vi "DDSSequence_BuildRamp.vi"(6 "Freqeuncy (MHz)":dbl[][](array[numeric]), 7 "Power":dbl[][](array[numeric]), 9 "Channels":T2(ring), 10 "Duration (ms)":dbl[][](array[numeric]), 11 "No of  active time blocks":dbl) -> (3 "appended instruction string":string)   [LabVIEW 2016]
panel:
  out "x/y":dbl
  in  "Ramp duration (us)":dbl=40.0 format="%#_6f"
  out "Step seperation (us)":dbl=0.4
  in  "Step Size":dbl=0.01 format="%#_6f"
  in  "Max Value":dbl=1.0 format="%#_13g"
  in  "Min Value":dbl format="%#_6f"
  in  "Ramp type":enum32{"Frequency", "Phase", "Amplitude"}(ring)=enum."Amplitude"
  in  "Ramp trigger source":T1(ring)=enum."BNC_IN_A_RISING"
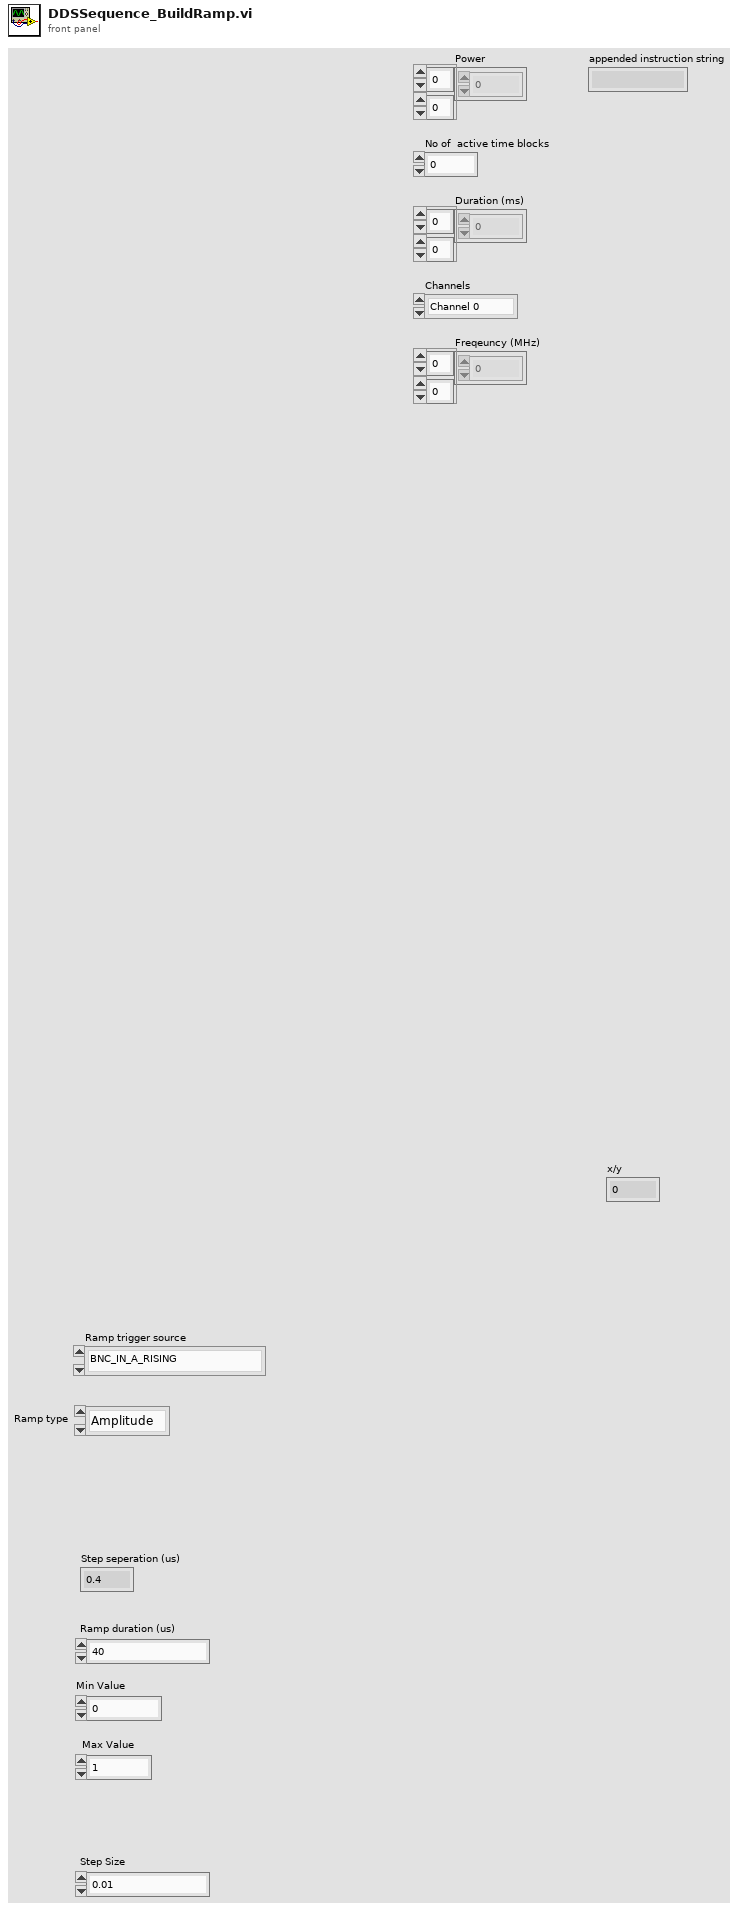
[diagram p1: front panel]
types:
  T1 = enum32{"O_RAMP_SWP_OVR", "RAM_SWP_OVR", "O_DROVER", "DROVER", "O_SPI_FIFO_EV1", "SPI_FIFO_EV1", "O_SPI_FIFO_EV0", "SPI_FIFO_EV0", "O_SPI_FIFO_FLUSHED", "SPI_FIFO_FLUSHED", "BNC_IN_B_LEVEL", "BNC_IN_B_FALLING", "BNC_IN_B_RISING", "BNC_IN_A_LEVEL", "BNC_IN_A_FALLING", "BNC_IN_A_RISING", "ALL_SPI_FIFOS_FLUSHED", "NONE"}
  T2 = enum32{"Channel 0", "Channel 1", "Both channels"}
  T3 = cluster{"Enable ASF from STP (F)":bool, "Digital ramp enable (F)":bool, "Digital ramp no-dwell high (F)":bool, "Digital ramp no-dwell low (F)":bool, "Matched latency enable (T)":bool, "Parallel data port enable (F)":bool}
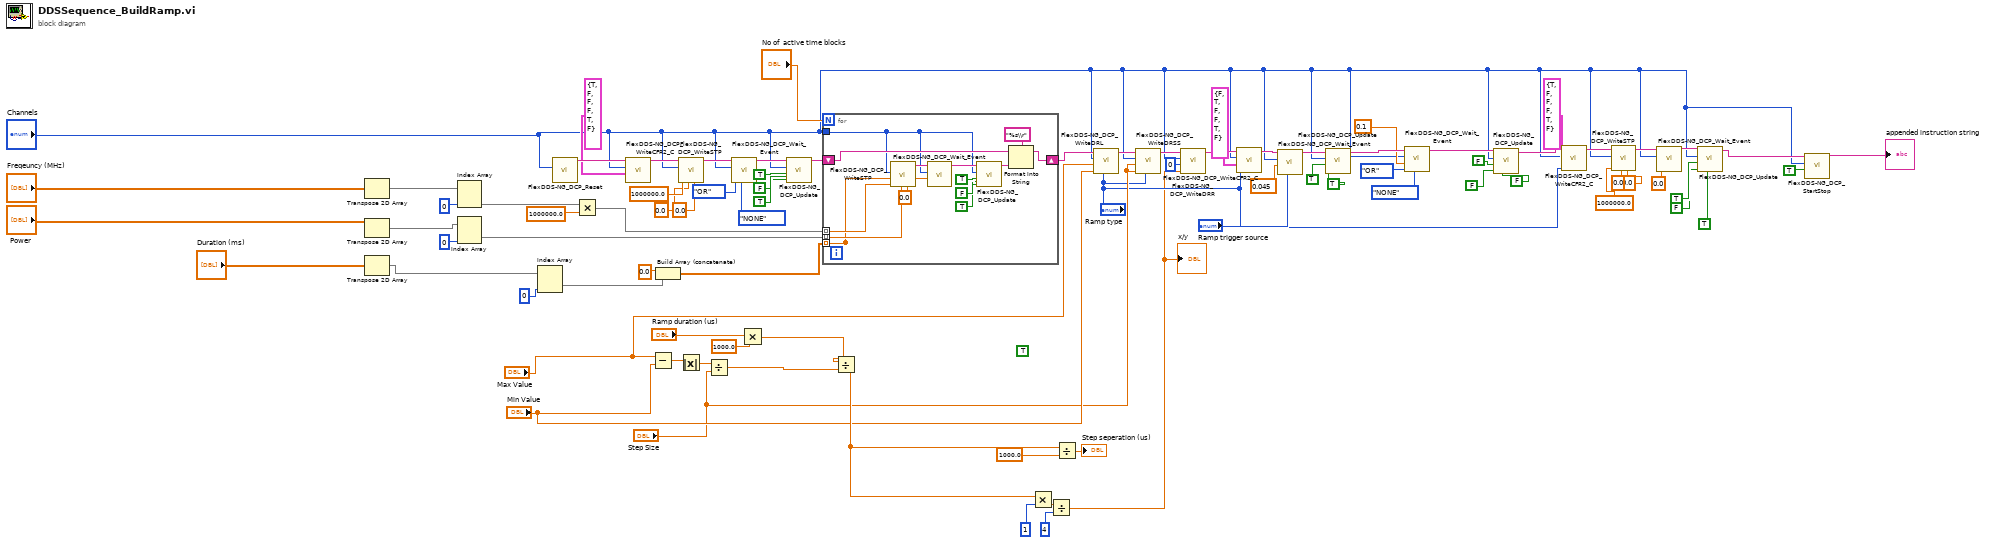
[diagram p0: block diagram]
diagram:
  (unwired) TRUE ("DRCTL(true=+, false=-) 2")
  n1 = Transpose 2D Array(2D array="Freqeuncy (MHz)") -> (transposed array=w74:dbl[][])
  n2 = Transpose 2D Array(2D array="Power") -> (transposed array=w71:dbl[][])
  n3 = Transpose 2D Array(2D array="Duration (ms)") -> (transposed array=w84:dbl[][])
  n4 = Index Array(array=w74, index (col)=0 ("index (row)")) -> (element=w76:dbl[])  [unwired: 1 in]
  n5 = Index Array(array=w71, index (col)=0 ("index (row)")) -> (element=w72:dbl[])  [unwired: 1 in]
  n6 = Index Array(array=w84, index (col)=0 ("index (row)")) -> (element=w81:dbl[])  [unwired: 1 in]
  n7 = call "FlexDDS-NG_DCP_Reset.vi"("Channels"="Channels") -> ("appended instruction string"=w56:string)  [unwired: 10 in]
  n8 = Multiply(x=w76, y=1000000.0 ("frequency Hz (0..400M)")) -> (x*y=w68:dbl[])
  n9 = call "FlexDDS-NG_DCP_WriteCFR2_C.vi"("CFR2 bits"=T3 {"Enable ASF from STP (F)"=TRUE, "Digital ramp enable (F)"=FALSE, "Digital ramp no-dwell high (F)"=FALSE, "Digital ramp no-dwell low (F)"=FALSE, "Matched latency enable (T)"=TRUE, "Parallel data port enable (F)"=FALSE} ("CFR2 bits 2"), "Channels"="Channels", "initial instruction string"=w56) -> ("appended instruction string"=w55:string)  [unwired: 8 in]
  n10 = Subtract(x="Max Value", y="Min Value") -> (x-y=w13:dbl)
  n11 = Build Array (concatenate)(0.0 ("phase degrees (0..360)"), w81) -> (w82:dbl[])
  n12 = call "FlexDDS-NG_DCP_WriteSTP.vi"("phase degrees (0..360)"=0.0, "amplitude (0..1)"=0.0, "frequency Hz (0..400M)"=1000000.0, "Channels"="Channels", "initial instruction string"=w55) -> ("appended instruction string"=w61:string)  [unwired: 6 in]
  n13 = Absolute Value(x=w13) -> (abs(x)=w12:dbl)
  n14 = Divide(x=w12, y="Step Size") -> (x/y=w17:dbl)
  n15 = call "FlexDDS-NG_DCP_Wait_Event.vi"("Event 1"=T1."NONE", "AND/OR"=enum32{"AND", "OR"}."OR", "Channels in"="Channels", "appended instruction string in"=w61) -> ("appended instruction string"=w60:string)  [unwired: 7 in]
  n16 = Multiply(x="Ramp duration (us)", y=1000.0) -> (x*y=w7:dbl)
  n17 = call "FlexDDS-NG_DCP_Update.vi"("ONLY IO_UPDATE"=TRUE, "DRCTL(true=+, false=-)"=FALSE ("DRCTL(true=+, false=-) 2"), "IO_UPDATE(true=u, false = '')"=TRUE ("IO_UPDATE(true=u, false = '')  2"), "Channels"="Channels", "appended instruction string in"=w60) -> ("appended instruction string out"=w66:string)  [unwired: 6 in]
  n18 = for {
    N: "No of  active time blocks" -> [_]
    shift-right: [w90] -> w24
    shift-left: w66 -> [w91]
    tunnel: w72 -> [w88] mode=indexing
    tunnel: "Channels" -> [w87]
    tunnel: w82 -> [w85] mode=indexing
    tunnel: w68 -> [w86] mode=indexing
    tunnel: [w85] -> _ mode=indexing
    n19 = call "FlexDDS-NG_DCP_WriteSTP.vi"("phase degrees (0..360)"=0.0, "amplitude (0..1)"=w88, "frequency Hz (0..400M)"=w86, "Channels"=w87) -> ("appended instruction string"=w93:string)  [unwired: 7 in]
    n20 = call "FlexDDS-NG_DCP_Wait_Event.vi"("waiting time [ms]"=w85, "Channels in"=w87, "appended instruction string in"=w93) -> ("appended instruction string"=w94:string)  [unwired: 8 in]
    n21 = call "FlexDDS-NG_DCP_Update.vi"("ONLY IO_UPDATE"=TRUE, "DRCTL(true=+, false=-)"=FALSE ("DRCTL(true=+, false=-) 2"), "IO_UPDATE(true=u, false = '')"=TRUE ("IO_UPDATE(true=u, false = '')  2"), "Channels"=w87, "appended instruction string in"=w94) -> ("appended instruction string out"=w89:string)  [unwired: 6 in]
    n22 = Format Into String(format string="%s\\r", initial string=w91, w89) -> (resulting string=w90:string)  [unwired: 1 in, 1 out]
  }
  n23 = Divide(x=w7, y=w17) -> (x/y=w16:dbl)
  n24 = Multiply(x=w16, y=u16 1) -> (x*y=w19:dbl)
  n25 = Divide(x=w19, y=u16 4) -> (x/y=w2:dbl)
  "x/y" <- w2
  n26 = Divide(x=w16, y=1000.0 ("x/y")) -> (x/y=→"Step seperation (us)":dbl)
  n27 = call "FlexDDS-NG_DCP_WriteDRL.vi"("Ramp type"="Ramp type", "low limit"="Min Value", "high limit"="Max Value", "Channels"="Channels", "initial instruction string"=w24) -> ("appended instruction string"=w51:string)  [unwired: 6 in]
  n28 = call "FlexDDS-NG_DCP_WriteDRSS.vi"("Ramp type"="Ramp type", "increment step size"="Step Size", "decrement step size"="Step Size", "Channels"="Channels", "initial instruction string"=w51) -> ("appended instruction string"=w50:string)  [unwired: 6 in]
  n29 = call "FlexDDS-NG_DCP_WriteDRR.vi"("digital ramp positive slope rate"=w2, "digital ramp negative slope rate"=u16 0, "Channels"="Channels", "initial instruction string"=w50) -> ("appended instruction string"=w49:string)  [unwired: 7 in]
  n30 = call "FlexDDS-NG_DCP_WriteCFR2_C.vi"("Digital ramp destination"="Ramp type", "CFR2 bits"=T3 {"Enable ASF from STP (F)"=FALSE, "Digital ramp enable (F)"=TRUE, "Digital ramp no-dwell high (F)"=FALSE, "Digital ramp no-dwell low (F)"=FALSE, "Matched latency enable (T)"=TRUE, "Parallel data port enable (F)"=FALSE}, "Channels"="Channels", "initial instruction string"=w49) -> ("appended instruction string"=w45:string)  [unwired: 7 in]
  n31 = call "FlexDDS-NG_DCP_Wait_Event.vi"("Event 1"="Ramp trigger source", "waiting time [ms]"=0.045, "Channels in"="Channels", "appended instruction string in"=w45) -> ("appended instruction string"=w44:string)  [unwired: 7 in]
  n32 = call "FlexDDS-NG_DCP_Update.vi"("DRCTL(true=+, false=-)"=TRUE, "IO_UPDATE(true=u, false = '')"=TRUE, "Channels"="Channels", "appended instruction string in"=w44) -> ("appended instruction string out"=w39:string)  [unwired: 7 in]
  n33 = call "FlexDDS-NG_DCP_Wait_Event.vi"("Event 1"=T1."NONE", "AND/OR"=enum32{"AND", "OR"}."OR", "waiting time [ms]"=0.1 ("y"), "Channels in"="Channels", "appended instruction string in"=w39) -> ("appended instruction string"=w27:string)  [unwired: 6 in]
  n34 = call "FlexDDS-NG_DCP_Update.vi"("ONLY IO_UPDATE"=FALSE, "DRCTL(true=+, false=-)"=FALSE ("DRCTL(true=+, false=-) 2"), "IO_UPDATE(true=u, false = '')"=FALSE ("IO_UPDATE(true=u, false = '')  2"), "Channels"="Channels", "appended instruction string in"=w27) -> ("appended instruction string out"=w28:string)  [unwired: 6 in]
  n35 = call "FlexDDS-NG_DCP_WriteCFR2_C.vi"("Digital ramp destination"="Ramp type", "CFR2 bits"=T3 {"Enable ASF from STP (F)"=TRUE, "Digital ramp enable (F)"=FALSE, "Digital ramp no-dwell high (F)"=FALSE, "Digital ramp no-dwell low (F)"=FALSE, "Matched latency enable (T)"=TRUE, "Parallel data port enable (F)"=FALSE}, "Channels"="Channels", "initial instruction string"=w28) -> ("appended instruction string"=w33:string)  [unwired: 7 in]
  n36 = call "FlexDDS-NG_DCP_WriteSTP.vi"("phase degrees (0..360)"=0.0, "amplitude (0..1)"=0.0, "frequency Hz (0..400M)"=1000000.0, "Channels"="Channels", "initial instruction string"=w33) -> ("appended instruction string"=w32:string)  [unwired: 6 in]
  n37 = call "FlexDDS-NG_DCP_Wait_Event.vi"("waiting time [ms]"=0.0, "Channels in"="Channels", "appended instruction string in"=w32) -> ("appended instruction string"=w31:string)  [unwired: 8 in]
  n38 = call "FlexDDS-NG_DCP_Update.vi"("ONLY IO_UPDATE"=TRUE, "DRCTL(true=+, false=-)"=FALSE ("DRCTL(true=+, false=-) 2"), "IO_UPDATE(true=u, false = '')"=TRUE ("IO_UPDATE(true=u, false = '')  2"), "Channels"="Channels", "appended instruction string in"=w31) -> ("appended instruction string out"=w23:string)  [unwired: 6 in]
  n39 = call "FlexDDS-NG_DCP_StartStop.vi"("start (T) stop (F)"=TRUE, "Channels"="Channels", "initial instruction string"=w23) -> ("appended instruction string"=→"appended instruction string":string)  [unwired: 8 in]
